vi "ziExample-AUXIn.vi"() -> ()   [LabVIEW 2009]
doc: "Control a Zurich instrument device via the LabOne Labview API. \nRequirements: Zurich Instruments MFLI, HF2 or UHFLI \nThis vi controls the aux outputs and reads the aux inputs.\n\n© Zurich Instruments AG, www.zhinst.com"
uses:
  <instrlib>/Zurich Instruments LabOne/Public/Data/ziTypeAuxInSample.ctl
  <instrlib>/Zurich Instruments LabOne/Public/Utility/ziTicksToS_vector.vi
  <instrlib>/Zurich Instruments LabOne/Public/Data/ziGetEventAuxInSample.vi
  <instrlib>/Zurich Instruments LabOne/Zurich Instruments LabOne.lvlib
panel:
  out "Error Out":errorcluster
  in  "Address":string="DEV"
  out "Selected Device":string
  in  "ramp":bool caption="Ramp Aux Out"
  in  "Samples":u32=1000
  out "Progress":dbl(slide) scale=0.0..1.0
  in  "stop":bool
  out "Waveform":cluster{dbl[], "Val Ch0 (V)":dbl[]}[](graph)
  # "Tested Instruments:\n- MFLI\n- HF2LI\n- UHFLI"
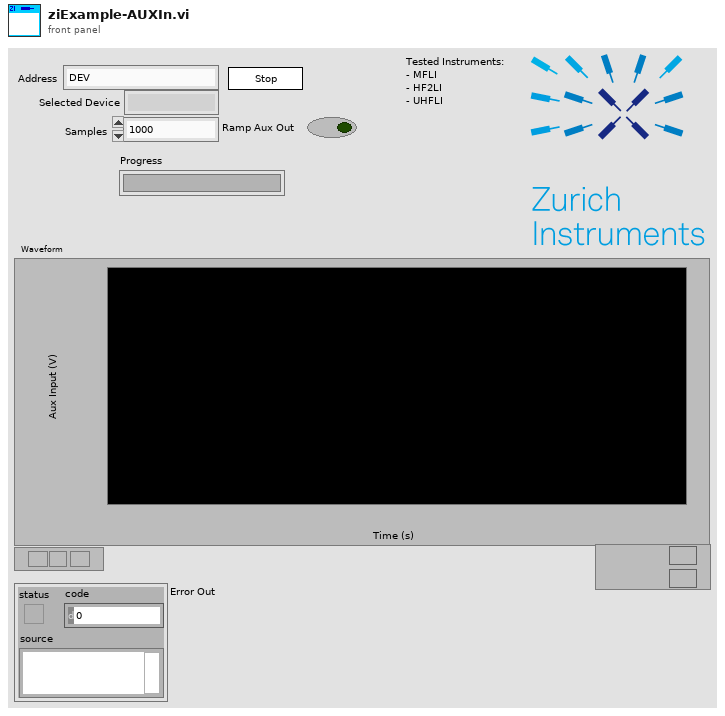
[diagram p1: front panel]
types:
  T1 = typedef "Zurich Instruments LabOne.lvlib/ziTypeAuxInSample.ctl" = cluster{"Timestamp (ticks)":u64[], "Val Ch0 (V)":dbl[], "Val Ch1 (V)":dbl[]}
  T2 = typedef "Zurich Instruments LabOne.lvlib/ziTypeHandle.ctl" = cluster{"handleValid":bool, "Conn":u64, "Path Prefix":string, "Handle":u64, "Connected":bool, "Clockbase(s)":dbl}
  T3 = typedef "Zurich Instruments LabOne.lvlib/ziTypePollType.ctl" = enum16{"NONE", "DOUBLE_DATA", "INTEGER_DATA", "DEMOD_SAMPLE", "SCOPE_WAVE_HF2", "AUXIN_SAMPLE", "DIO_SAMPLE", "BYTE_ARRAY", "PWA_WAVE", "9", "10", "11", "12", "13", "14", "15", "TREE_CHANGE_DEPRI", "17", "ERROR", "19", "20", "21", "22", "23", "24", "25", "26", "27", "28", "29", "30", "31", "DOUBLE_DATA_TS", "INTEGER_DATA_TS", "34", "SCOPE_WAVE", "SCOPE_WAVE_EX", "37", "BYTE_ARRAY_TS", "39", "40", "41", "42", "43", "44", "45", "CNT_DATA", "47", "TREE_CHANGE", "49", "50", "51", "52", "53", "54", "55", "56", "57", "58", "59", "60", "61", "62", "63", "SWEEPER_DATA", "SPECTRUM_DATA", "ADVISOR_DATA", "VECTOR_DATA", "IMP_DATA"}
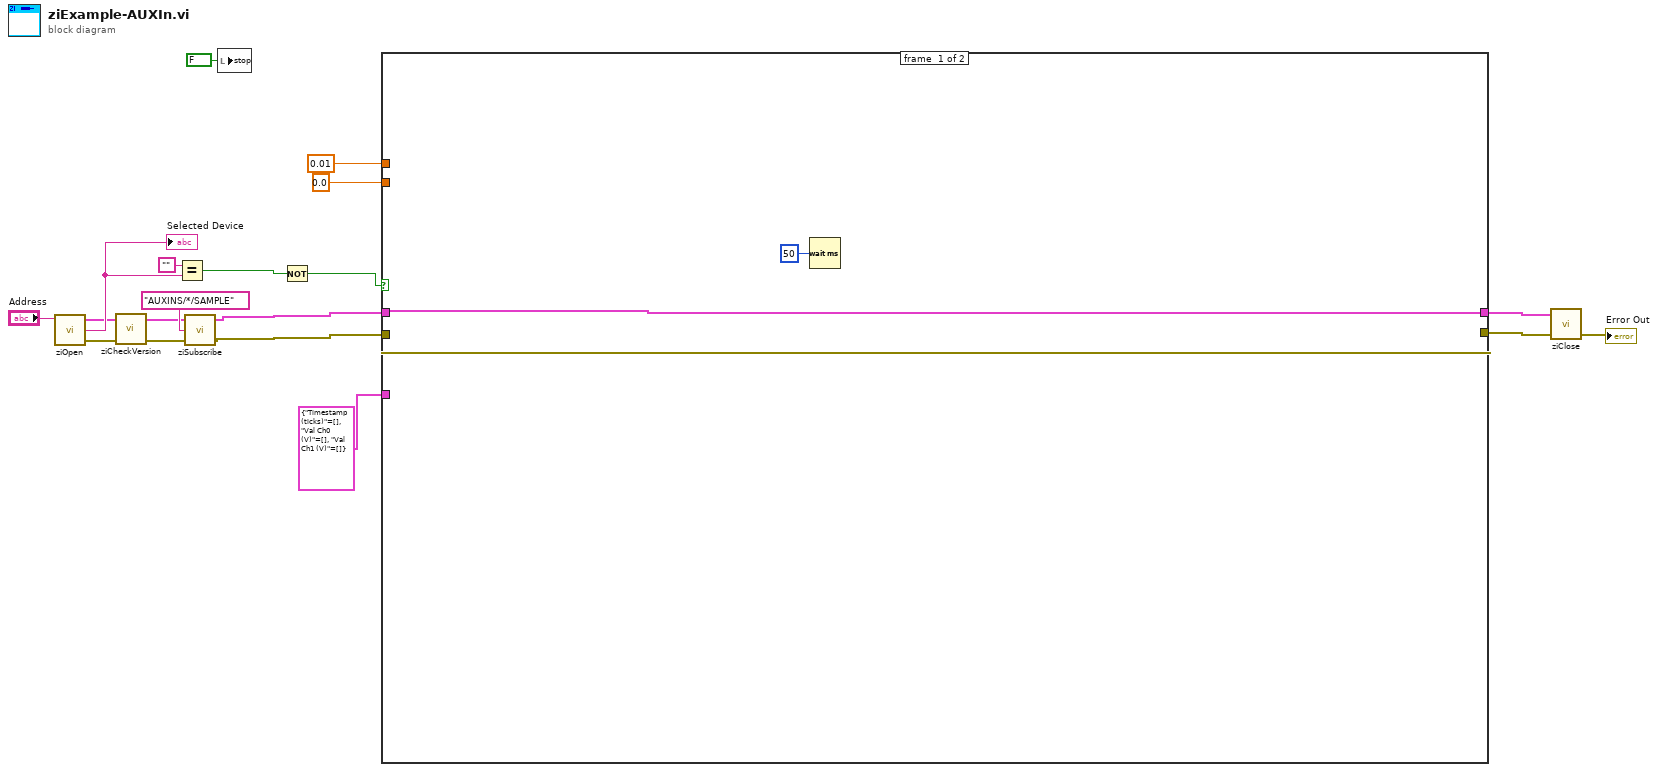
[diagram p0: block diagram]
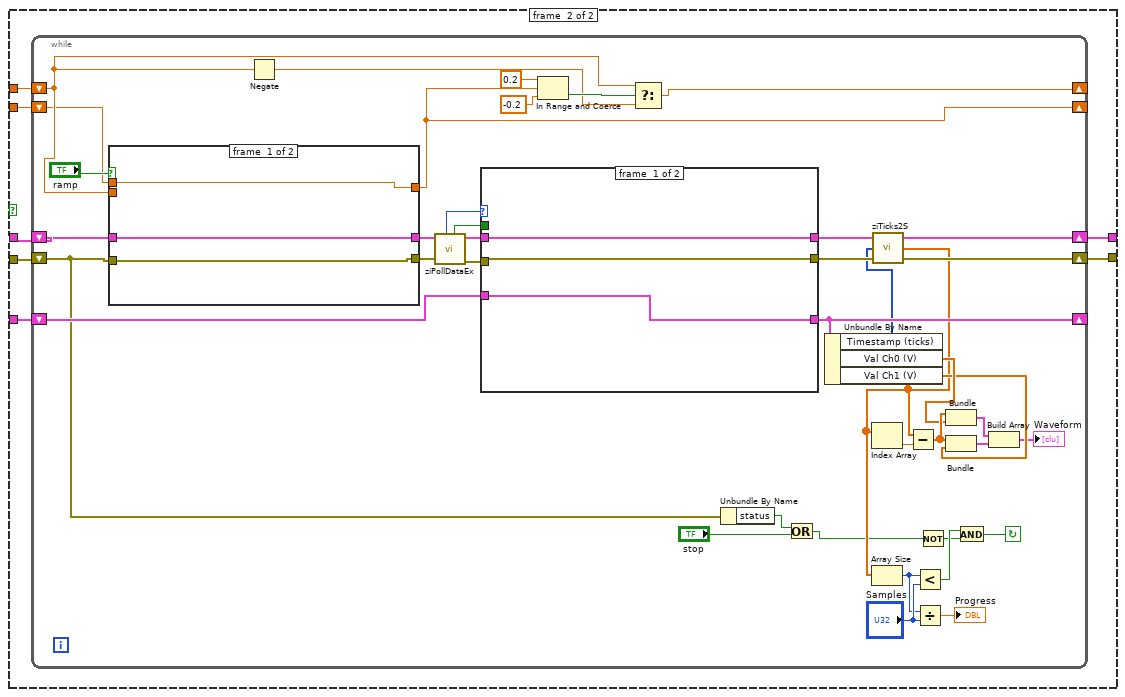
[diagram p2: hidden frame]
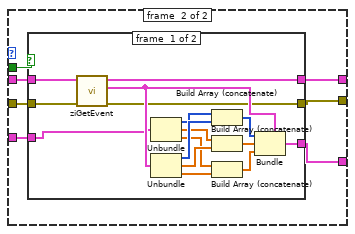
[diagram p3: hidden frame]
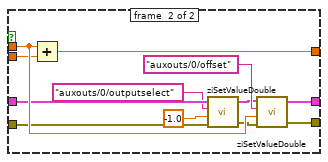
[diagram p5: hidden frame]
diagram:
  n1 = call <instrlib>:"ziOpen.vi"("Address"="Address") -> ("Error Out"=w7:errorcluster, "Selected Device"=w15:string, "HandleOut"=w8:T2)  [unwired: 1 in, 2 out]
  "Selected Device" <- w15
  n2 = call <instrlib>:"ziCheckVersion.vi"("Handle In"=w8, "Error In"=w7) -> ("Handle Out"=w5:T2, "Error Out"=w6:errorcluster)  [unwired: 11 in, 1 out]
  n3 = Equal?(x="", y=w15) -> (x = y?=w9:bool)
  n4 = call <instrlib>:"ziSubscribe.vi"("error in"=w6, "Path ()"="AUXINS/*/SAMPLE", "Handle In"=w5) -> ("error out"=w10:errorcluster, "Handle Out"=w11:T2)  [unwired: 1 out]
  n5 = local write "stop"(FALSE ("run")) -> ()
  n6 = Not(x=w9) -> (.not. x?=w1:bool)
  n7 = case shown="True" w1 {
    tunnel: [w21 w29] -> w17
    tunnel: [w20 w28] -> w16
    tunnel: w11 -> [w20 w27]
    tunnel: w10 -> [w21 w26]
    tunnel: T1 {"Timestamp (ticks)"=[], "Val Ch0 (V)"=[], "Val Ch1 (V)"=[]} ("AuxIn Out") -> [_ w25]
    tunnel: 0.01 -> [_ w24]
    tunnel: 0.0 -> [_ w23]
    frame #0 {
      n8 = Wait (ms)(milliseconds to wait=50) -> ()  [unwired: 1 out]
    }
    frame #1 {
      n9 = while {
        shift-right: [w46] -> w28
        shift-left: w27 -> [w68]
        shift-right: [w47] -> w29
        shift-left: w26 -> [w30]
        shift-right: [w50] -> _
        shift-left: w25 -> [w51]
        shift-right: [w37] -> _
        shift-left: w24 -> [w36]
        shift-right: [w34] -> _
        shift-left: w23 -> [w35]
        stop <- w60 continue-if-true
        n10 = case shown="True" "ramp" {
          tunnel: w30 -> [w101 w108]
          tunnel: w68 -> [w100 w109]
          tunnel: w35 -> [w102 w113]
          tunnel: w36 -> [_ w103]
          tunnel: [w102 w112] -> w34
          tunnel: [w101 w111] -> w67
          tunnel: [w100 w110] -> w66
          frame #0 {
          }
          frame #1 {
            n11 = Add(x=w113, y=w103) -> (x+y=w112:dbl)
            n12 = call <instrlib>:"ziSetValueDouble.vi"("Error In"=w108, "Value"=-1.0, "Path"="auxouts/0/outputselect", "Handle In"=w109) -> ("Error Out"=w107:errorcluster, "Handle Out"=w106:T2)  [unwired: 1 out]
            n13 = call <instrlib>:"ziSetValueDouble.vi"("Error In"=w107, "Value"=w113, "Path"="auxouts/0/offset", "Handle In"=w106) -> ("Error Out"=w111:errorcluster, "Handle Out"=w110:T2)  [unwired: 1 out]
          }
        }
        n14 = Negate(x=w36) -> (-x=w54:dbl)
        n15 = call <instrlib>:"ziPollDataEx.vi"("error in"=w67, "Handle In"=w66) -> ("error out"=w61:errorcluster, "Handle Out"=w62:T2, "Timed Out"=w70:bool, "ziValueType"=w58:T3)  [unwired: 2 in, 4 out]
        n16 = case shown="\"AUXIN_SAMPLE\"" w58 {
          tunnel: w70 -> [_ w80]
          tunnel: w62 -> [w73 w79]
          tunnel: [w73 w78] -> w49
          tunnel: w61 -> [w72 w77]
          tunnel: [w72 w76] -> w48
          tunnel: [w71 w75] -> w50
          tunnel: w51 -> [w71 w74]
          frame #0 {
          }
          frame #1 {
            n17 = case shown="False" w80 {
              tunnel: w79 -> [w96 w99]
              tunnel: [w87 w99] -> w78
              tunnel: w77 -> [w95 w98]
              tunnel: [w88 w98] -> w76
              tunnel: [w85 w97] -> w75
              tunnel: w74 -> [w84 w97]
              frame #0 {
                n18 = call-poly <instrlib>:"ziGetEvent.vi"("Error In"=w95, "Handle In"=w96) -> ("Error Out"=w88:errorcluster, "AuxIn Out"=w92:T1, "Handle Out"=w87:T2)  [unwired: 7 in]
                n19 = Unbundle(w84) -> ("Timestamp (ticks)"=w81:u64[], "Val Ch0 (V)"=w83:dbl[], "Val Ch1 (V)"=w82:dbl[])
                n20 = Unbundle(w92) -> ("Timestamp (ticks)"=w86:u64[], "Val Ch0 (V)"=w93:dbl[], "Val Ch1 (V)"=w94:dbl[])
                n21 = Build Array (concatenate)(w81, w86) -> (w91:u64[])
                n22 = Build Array (concatenate)(w83, w93) -> (w90:dbl[])
                n23 = Build Array (concatenate)(w82, w94) -> (w89:dbl[])
                n24 = Bundle(cluster=w92, "Timestamp (ticks)"=w91, "Val Ch0 (V)"=w90, "Val Ch1 (V)"=w89) -> (w85:T1)
              }
              frame #1 {
              }
            }
          }
        }
        n25 = In Range and Coerce(upper limit=0.2 ("y"), x=w34, lower limit=-0.2 ("y")) -> (In Range?=w55:bool)  [unwired: 1 out]
        n26 = Select(t=w36, s=w55, f=w54) -> (s? t:f=w37:dbl)
        n27 = Unbundle By Name(w30) -> ("status"=w32:bool)
        n28 = Or(x=w32, y="stop") -> (x .or. y?=w31:bool)
        n29 = Unbundle By Name(w50) -> ("Timestamp (ticks)"=w45:u64[], "Val Ch0 (V)"=w44:dbl[], "Val Ch1 (V)"=w43:dbl[])
        n30 = call-poly <instrlib>:"ziTicks2S.vi"("Error In"=w48, "Timestamp (ticks)"=w45, "Handle In"=w49) -> ("Error Out"=w47:errorcluster, "Timestamp(s)"=w40:dbl[], "Handle Out"=w46:T2)
        n31 = Index Array(array=w40) -> (element=w41:dbl)  [unwired: 1 in]
        n32 = Array Size(array=w40) -> (size(s)=w64:i32)
        n33 = Subtract(x=w40, y=w41) -> (x-y=w53:dbl[])
        n34 = Less?(x=w64, y="Samples") -> (x < y?=w69:bool)
        n35 = Divide(x=w64, y="Samples") -> (x/y=→"Progress":dbl)
        n36 = Not(x=w31) -> (.not. x?=w59:bool)
        n37 = Bundle(w53, "Val Ch0 (V)"=w44) -> (w52:cluster{dbl[], "Val Ch0 (V)":dbl[]})  [unwired: 1 out]
        n38 = Bundle(w53, "Val Ch1 (V)"=w43) -> (w42:cluster{dbl[], "Val Ch1 (V)":dbl[]})  [unwired: 1 out]
        n39 = And(x=w69, y=w59) -> (x .and. y?=w60:bool)
        n40 = Build Array(w52, w42) -> (→"Waveform":cluster{dbl[], "Val Ch1 (V)":dbl[]}[])
      }
    }
  }
  n41 = call <instrlib>:"ziClose.vi"("Error In"=w17, "Handle In"=w16) -> ("Error Out"=→"Error Out":errorcluster)  [unwired: 3 out]
